vi "myo_vibrate_simple.vi"(6 "Connection Status":T1={"MAC Address"="", "cnx handle"=0, "cnx flags"=0, "Address Type"=125, "Connection Interval (ms)"=125, "Timeout(ms)"=125, "Latency"=0, "bonding handle"=0} {"Address Type" items=["Public", "Random"]}, 8 "error in (no error)":errorcluster, 10 "Handle table":string[][](array[string]), 11 "VISA Refnum in":refnum<visa-resource-name>) -> (0 "error out":errorcluster, 3 "VISA Refnum out":refnum<visa-resource-name>)   [LabVIEW 2013]
uses:
  code/labview/bluetooth_le/bluegiga/type_def/connection_status_bundle.ctl
  code/labview/bluetooth_le/bluegiga/type_def/address_type.ctl
  code/labview/bluetooth_le/bluegiga/functions/ble_write_by_service_characteristic_uint8array.vi
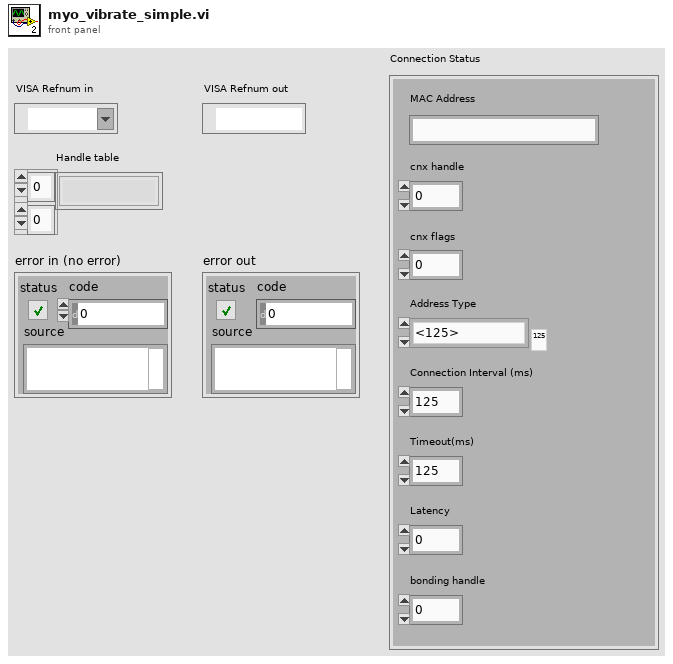
[diagram p1: front panel]
types:
  T1 = typedef "connection_status_bundle.ctl" = cluster{"MAC Address":string, "cnx handle":u8, "cnx flags":u8, "Address Type":T2, "Connection Interval (ms)":u16, "Timeout(ms)":u16, "Latency":u16, "bonding handle":u8}
  T2 = typedef "address_type.ctl" = u8
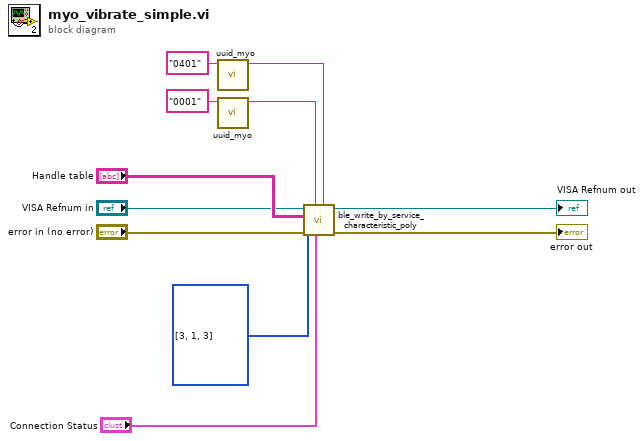
[diagram p0: block diagram]
diagram:
  n1 = call "uuid_myo.vi"("MYO  UUID (16bits)"="0401") -> ("full UUID"=w4:string)  [unwired: 10 in]
  n2 = call "uuid_myo.vi"("MYO  UUID (16bits)"="0001") -> ("full UUID"=w5:string)  [unwired: 10 in]
  n3 = call-poly "ble_write_by_service_characteristic_poly.vi"("Characteristic UUID"=w4, "Connection Status"="Connection Status", "Service UUID"=w5, "error in (no error)"="error in (no error)", "data"=u8[] [3, 1, 3], "Handle table"="Handle table", "COM Bluegiga in"="VISA Refnum in") -> ("error out"=→"error out":errorcluster, "COM Bluegiga out"=→"VISA Refnum out":refnum<visa-resource-name>)  [unwired: 3 in]
